vi "PathPlanner_PathSegment_New.vi"(5 "P1":T5 {"Y" format="%14.3f"; "X" format="%14.3f"}, 6 "EndSegment":bool, 7 "P2":T5 {"Y" format="%14.3f"; "X" format="%14.3f"}, 8 "ConstraintZones":T1[](array[typedef]), 9 "TargetHolonomicRotations":T3[](array[typedef]) {"target"."SIN" format="%13.4f"; "target"."COS" format="%13.4f"; "target"."VALUE" format="%13.4f"}, 10 "P4":T5 {"Y" format="%14.3f"; "X" format="%14.3f"}, 11 "P3":T5 {"Y" format="%14.3f"; "X" format="%14.3f"}) -> (3 "Segment":T6 {"SegmentPoints"."HolonomicRotation"."SIN" format="%13.4f"; "SegmentPoints"."HolonomicRotation"."COS" format="%13.4f"; "SegmentPoints"."HolonomicRotation"."VALUE" format="%13.4f"; "SegmentPoints"."Position"."Y" format="%14.3f"; "SegmentPoints"."Position"."X" format="%14.3f"})   [LabVIEW 2019, in "PathPlanner24.lvlib"]
doc: "Generate a new path segment\n\nInputs: \n - p1 - translation2d - Start anchor point\n - p2 - translation2d - Start next control\n - p3 - translation2d - End prev control\n - p4 - translation2d - End anchor point\n - targetHolonomicRotations - array Rotation targets for within this segment (Optional. Default: empty)\n - constraintZones - array - Constraint zones for within this segment (Optional. Default: empty)\n - endSegment - boolean - Is this the last segment in the path\n\nOutputs:\n - Segment - cluster - Data defining path segment"
uses:
  PathPlanner24.lvlib
  TypeDef/PathPlannerPathSegment.ctl
  TypeDef/PathPlannerPathPoint.ctl
  <vilib>/Rock Robotics/WPI/ThirdParty/JAS_Junk/TrajLib/TypeDef/TRANSLATION2D.ctl
  <vilib>/Rock Robotics/WPI/ThirdParty/JAS_Junk/TrajLib/TypeDef/ROTATION2D.ctl
  TypeDef/PathPlannerPathConstraints.ctl
  TypeDef/PathPlannerRotationTarget.ctl
  TypeDef/PathPlannerConstraintsZone.ctl
  PathPlanner_ConstraintsZone_IsWithinZone.vi
  <vilib>/Rock Robotics/WPI/ThirdParty/JAS_Junk/TrajLib/Trajectory_Library.lvlib
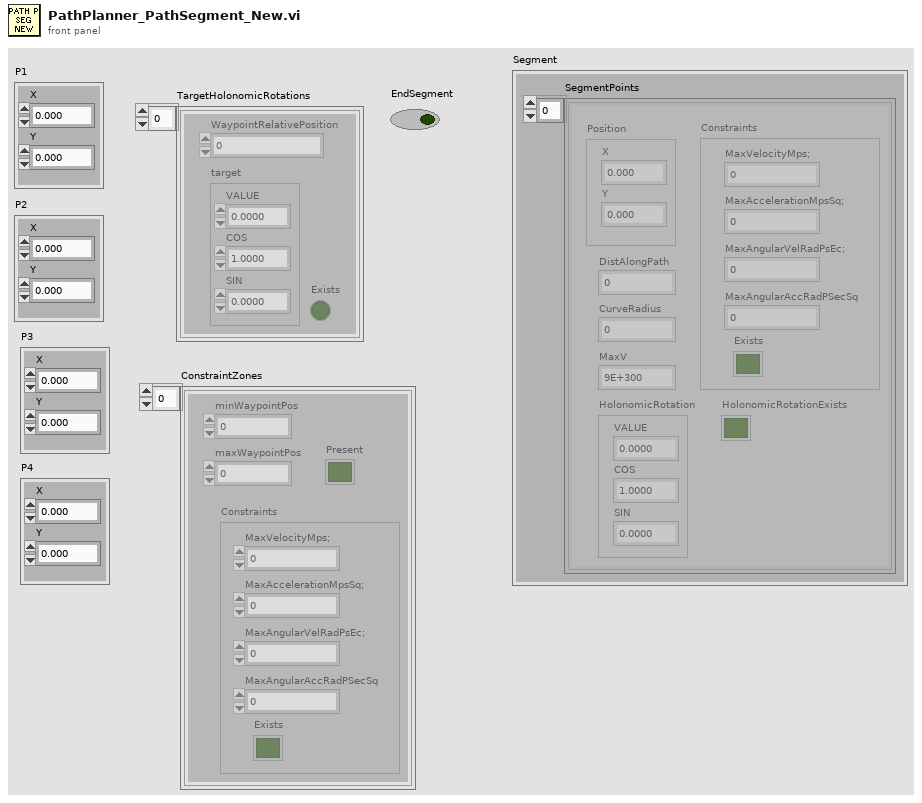
[diagram p1: front panel]
types:
  T1 = typedef "PathPlanner24.lvlib/PathPlannerConstraintsZone.ctl" = cluster{"minWaypointPos":dbl, "maxWaypointPos":dbl, "Constraints":T2, "Present":bool}
  T2 = typedef "PathPlanner24.lvlib/PathPlannerPathConstraints.ctl" = cluster{"MaxVelocityMps;":dbl, "MaxAccelerationMpsSq;":dbl, "MaxAngularVelRadPsEc;":dbl, "MaxAngularAccRadPSecSq":dbl, "Exists":bool}
  T3 = typedef "PathPlanner24.lvlib/PathPlannerRotationTarget.ctl" = cluster{"target":T4, "WaypointRelativePosition":dbl, "Exists":bool}
  T4 = typedef "Trajectory_Library.lvlib/ROTATION2D.ctl" = cluster{"VALUE":dbl, "COS":dbl, "SIN":dbl}
  T5 = typedef "Trajectory_Library.lvlib/TRANSLATION2D.ctl" = cluster{"X":dbl, "Y":dbl}
  T6 = typedef "PathPlanner24.lvlib/PathPlannerPathSegment.ctl" = cluster{"SegmentPoints":T7[]}
  T7 = typedef "PathPlanner24.lvlib/PathPlannerPathPoint.ctl" = cluster{"Position":T5, "HolonomicRotation":T4, "DistAlongPath":dbl, "CurveRadius":dbl, "MaxV":dbl, "Constraints":T2, "HolonomicRotationExists":bool}
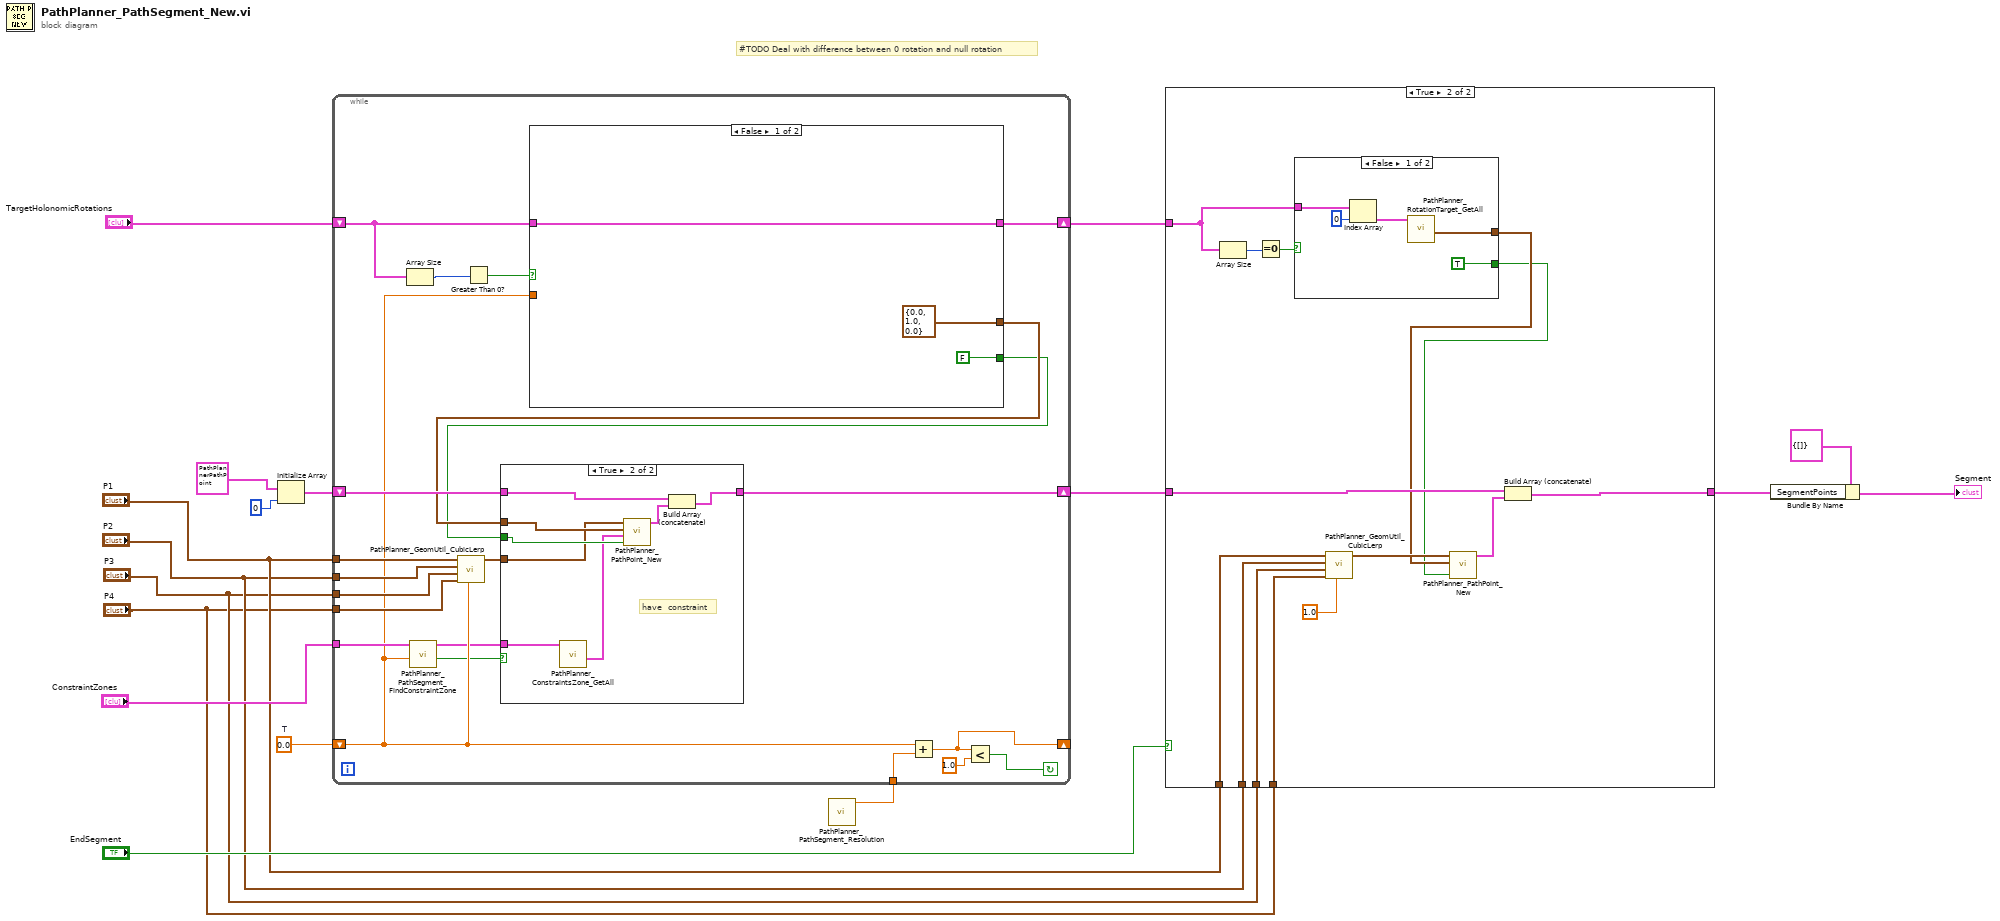
[diagram p0: block diagram]
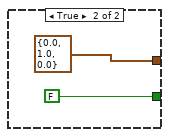
[diagram p3: hidden frame]
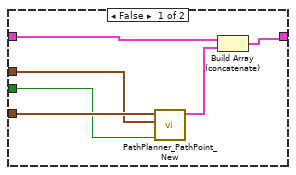
[diagram p4: hidden frame]
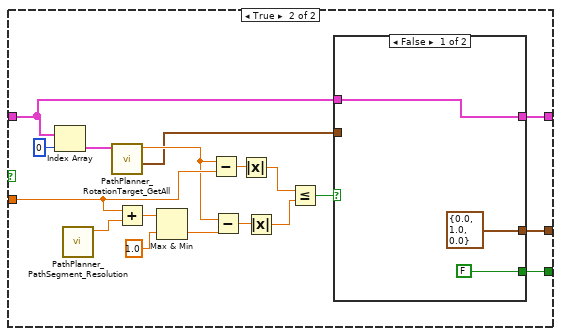
[diagram p5: hidden frame]
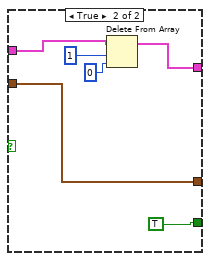
[diagram p6: hidden frame]
diagram:
  w15 = 0.0  # T
  # "#TODO Deal with difference between 0 rotation and null rotation"
  n1 = Initialize Array(T7 {"Position"={"X"=0.0, "Y"=0.0}, "HolonomicRotation"={"VALUE"=0.0, "COS"=1.0, "SIN"=0.0}, "DistAlongPath"=0.0, "CurveRadius"=0.0, "MaxV"=9e+300, "Constraints"={"MaxVelocityMps;"=0.0, "MaxAccelerationMpsSq;"=0.0, "MaxAngularVelRadPsEc;"=0.0, "MaxAngularAccRadPSecSq"=0.0, "Exists"=FALSE}, "HolonomicRotationExists"=FALSE} ("PathPlannerPoint"), 0 ("dimension size")) -> (w11:T7[])
  n2 = call "PathPlanner_PathSegment_Resolution.vi"() -> ("Resolution"=w14:dbl)  [unwired: 11 in]
  n3 = while {
    shift-right: [w36] -> _
    shift-left: w15 -> [w25]
    tunnel: w14 -> [w38]
    tunnel: "ConstraintZones" -> [w32]
    shift-right: [w33] -> w5
    shift-left: "TargetHolonomicRotations" -> [w34]
    shift-right: [w26] -> w9
    shift-left: w11 -> [w31]
    tunnel: "P1" -> [w30]
    tunnel: "P2" -> [w29]
    tunnel: "P3" -> [w28]
    tunnel: "P4" -> [w27]
    stop <- w35 continue-if-true
    n4 = Array Size(array=w34) -> (size(s)=w19:i32)
    n5 = call "PathPlanner_PathSegment_FindConstraintZone.vi"("T"=w25, "Zones"=w32) -> ("IsPresent"=w20:bool, "Returned Zone"=w22:T1)  [unwired: 8 in]
    n6 = call "PathPlanner_GeomUtil_CubicLerp.vi"("T"=w25, "D"=w27, "C"=w28, "B"=w29, "A"=w30) -> ("Lerp"=w21:T5)  [unwired: 6 in]
    n7 = Greater Than 0?(x=w19) -> (x > 0?=w18:bool)
    n8 = case shown="False" w18 {
      tunnel: w34 -> [w55 w58]
      tunnel: [w55 w57] -> w33
      tunnel: w25 -> [_ w69]
      tunnel: [T4 {"VALUE"=0.0, "COS"=1.0, "SIN"=0.0} ("ROTATION") w60] -> w24
      tunnel: [FALSE w56] -> w23
      frame False {
      }
      frame True {
        n9 = Index Array(array=w58, index=0) -> (element=w72:T3)
        n10 = call "PathPlanner_PathSegment_Resolution.vi"() -> ("Resolution"=w70:dbl)  [unwired: 11 in]
        n11 = call "PathPlanner_RotationTarget_GetAll.vi"("RotationTarget"=w72) -> ("target"=w59:T4, "WaypointRelativePosition"=w65:dbl)  [unwired: 8 in, 1 out]
        n12 = Add(x=w69, y=w70) -> (x+y=w68:dbl)
        n13 = Max & Min(x=w68, y=1.0) -> (min(x,y)=w66:dbl)  [unwired: 1 out]
        n14 = Subtract(x=w65, y=w69) -> (x-y=w71:dbl)
        n15 = Subtract(x=w65, y=w66) -> (x-y=w64:dbl)
        n16 = Absolute Value(x=w71) -> (abs(x)=w62:dbl)
        n17 = Absolute Value(x=w64) -> (abs(x)=w63:dbl)
        n18 = Less Or Equal?(x=w62, y=w63) -> (x <= y?=w61:bool)
        n19 = case shown="False" w61 {
          tunnel: [T4 {"VALUE"=0.0, "COS"=1.0, "SIN"=0.0} ("ROTATION") w82] -> w60
          tunnel: w59 -> [_ w82]
          tunnel: w58 -> [w75 w81]
          tunnel: [w75 w78] -> w57
          tunnel: [FALSE TRUE] -> w56
          frame False {
          }
          frame True {
            n20 = Delete From Array(array=w81, length=1, index=0) -> (array with subset deleted=w78:T3[])  [unwired: 1 out]
          }
        }
      }
    }
    n21 = case shown="True" w20 {
      tunnel: w31 -> [w43 w52]
      tunnel: [w42 w51] -> w26
      tunnel: w24 -> [w40 w50]
      tunnel: w23 -> [w39 w49]
      tunnel: w22 -> [_ w48]
      tunnel: w21 -> [w41 w46]
      frame False {
        n22 = call "PathPlanner_PathPoint_New.vi"("Rotation\nExists"=w39, "HolonomicRotation"=w40, "Position"=w41) -> ("PathPlannerPoint"=w44:T7)  [unwired: 8 in]
        n23 = Build Array (concatenate)(w43, w44) -> (w42:T7[])
      }
      frame True {
        # "have  constraint"
        n24 = call "PathPlanner_ConstraintsZone_GetAll.vi"("ConstraintsZone"=w48) -> ("Constraints"=w45:T2)  [unwired: 8 in, 2 out]
        n25 = call "PathPlanner_PathPoint_New.vi"("Rotation\nExists"=w49, "Constraints"=w45, "HolonomicRotation"=w50, "Position"=w46) -> ("PathPlannerPoint"=w47:T7)  [unwired: 7 in]
        n26 = Build Array (concatenate)(w52, w47) -> (w51:T7[])
      }
    }
    n27 = Add(x=w25, y=w38) -> (x+y=w36:dbl)
    n28 = Less?(x=w36, y=1.0) -> (x < y?=w35:bool)
  }
  n29 = case shown="True" "EndSegment" {
    tunnel: w9 -> [w83 w89]
    tunnel: [w83 w88] -> w6
    tunnel: w5 -> [_ w95]
    tunnel: "P1" -> [_ w94]
    tunnel: "P2" -> [_ w87]
    tunnel: "P3" -> [_ w93]
    tunnel: "P4" -> [_ w92]
    frame False {
    }
    frame True {
      n30 = Array Size(array=w95) -> (size(s)=w97:i32)
      n31 = Equal To 0?(x=w97) -> (x = 0?=w96:bool)
      n32 = case shown="False" w96 {
        tunnel: w95 -> [w101 _]
        tunnel: [w99 T4 {"VALUE"=0.0, "COS"=1.0, "SIN"=0.0} ("ROTATION")] -> w85
        tunnel: [TRUE FALSE] -> w84
        frame False {
          n33 = Index Array(array=w101, index=0) -> (element=w100:T3)
          n34 = call "PathPlanner_RotationTarget_GetAll.vi"("RotationTarget"=w100) -> ("target"=w99:T4)  [unwired: 8 in, 2 out]
        }
        frame True {
        }
      }
      n35 = call "PathPlanner_GeomUtil_CubicLerp.vi"("T"=1.0, "D"=w92, "C"=w93, "B"=w87, "A"=w94) -> ("Lerp"=w86:T5)  [unwired: 6 in]
      n36 = call "PathPlanner_PathPoint_New.vi"("Rotation\nExists"=w84, "HolonomicRotation"=w85, "Position"=w86) -> ("PathPlannerPoint"=w90:T7)  [unwired: 8 in]
      n37 = Build Array (concatenate)(w89, w90) -> (w88:T7[])
    }
  }
  n38 = Bundle By Name(cluster=T6 {"SegmentPoints"=[]} ("Segment"), "SegmentPoints"=w6) -> (→"Segment":T6)
